vi "CRYProject Editor PIC Action Start.vi"(10 "sData":string) -> ()   [LabVIEW 2013]
uses:
  CRYProject Editor Global.vi
  CRYWindow/SubVI/CRYMain Sub Window Global.vi
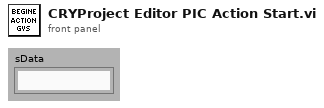
[diagram p1: front panel]
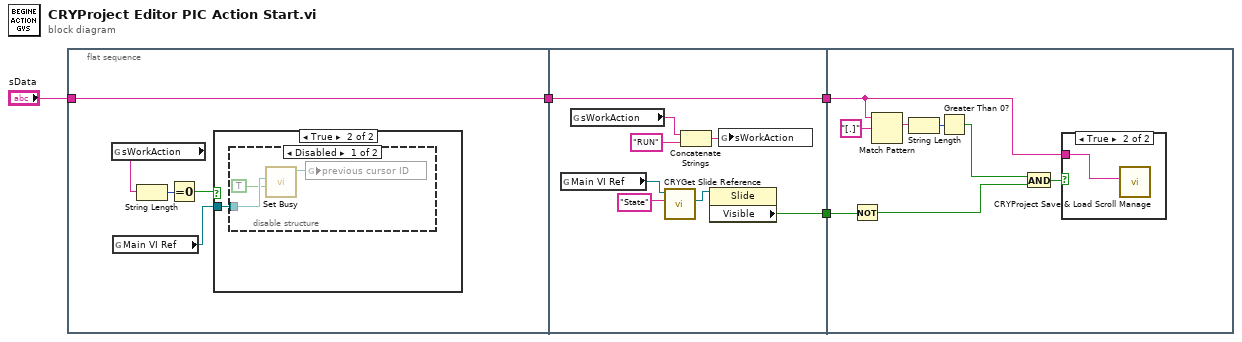
[diagram p0: block diagram]
diagram:
  n1 = flat-sequence {
    tunnel: "sData" -> [w9]
    tunnel: [w9] -> w1
    tunnel: [w21] -> w3
    tunnel: [w15] -> w2
    tunnel: w1 -> [w21]
    tunnel: w3 -> [w27]
    tunnel: w2 -> [w29]
    frame #0 {
      n2 = global read "CRYProject Editor Global.vi" "sWorkAction"() -> (w8:string)
      n3 = global read "CRYMain Sub Window Global.vi" "Main VI Ref"() -> (w5:refnum<vi>)
      n4 = String Length(string=w8) -> (length=w7:i32)
      n5 = Equal To 0?(x=w7) -> (x = 0?=w6:bool)
      n6 = case shown="True" w6 {
        tunnel: w5 -> [_ w10]
        frame False {
        }
        frame True {
          n7 = disable-structure shown="Disabled" {
            disable-tunnel: w10 -> [w13 _]
            frame Disabled {
              n8 = call <vilib>:"Set Busy.vi"("disable click? (T)"=TRUE, "VI reference (current VI)"=w13) -> ("previous cursor ID"=w11:refnum<k1>)  [unwired: 8 in, 1 out]
              n9 = global write "CRYProject Editor Global.vi" "previous cursor ID"(w11) -> ()
            }
            frame Enabled {
            }
          }
        }
      }
    }
    frame #1 {
      n10 = global read "CRYMain Sub Window Global.vi" "Main VI Ref"() -> (w14:refnum<vi>)
      n11 = global read "CRYProject Editor Global.vi" "sWorkAction"() -> (w19:string)
      n12 = call "CRYGet Slide Reference.vi"("Label Name"="State" ("Type"), "VI Refnum"=w14) -> ("Slide Ref Out"=w17:refnum<vi>)  [unwired: 9 out]
      n13 = Concatenate Strings(w19, "RUN" ("string")) -> (w20:string)
      n14 = property class="Slide"(reference=w17) -> ("Visible"=w15:bool)  [unwired: 1 in, 2 out]
      n15 = global write "CRYProject Editor Global.vi" "sWorkAction"(w20) -> ()
    }
    frame #2 {
      n16 = Not(x=w29) -> (.not. x?=w23:bool)
      n17 = Match Pattern(string=w27, regular expression="[.]") -> (match substring=w25:string)  [unwired: 1 in, 3 out]
      n18 = String Length(string=w25) -> (length=w24:i32)
      n19 = Greater Than 0?(x=w24) -> (x > 0?=w22:bool)
      n20 = And(x=w22, y=w23) -> (x .and. y?=w28:bool)
      n21 = case shown="True" w28 {
        tunnel: w27 -> [_ w30]
        frame False {
        }
        frame True {
          n22 = call "CRYProject Save & Load Scroll Manage.vi"("StateLabel"=w30) -> ()  [unwired: 11 in]
        }
      }
    }
  }
